vi "refmgr_register.vi"(8 "error in (no error)":errorcluster, 9 "ViName":string, 10 "VI Refnum":refnum<vi>, 11 "TagDB in":T1) -> (0 "error out":errorcluster, 2 "VI Refnum (dup)":refnum<vi>, 3 "TagDB out":T1)   [LabVIEW 2014, in "RefManager(dev).lvlib"]
uses:
  RefManager(dev).lvlib
  <userlib>/_NEVSTOP/TagDB/Core/tagDB_Def.ctl
  <userlib>/_NEVSTOP/TagDB/Core/TagDB.lvlib
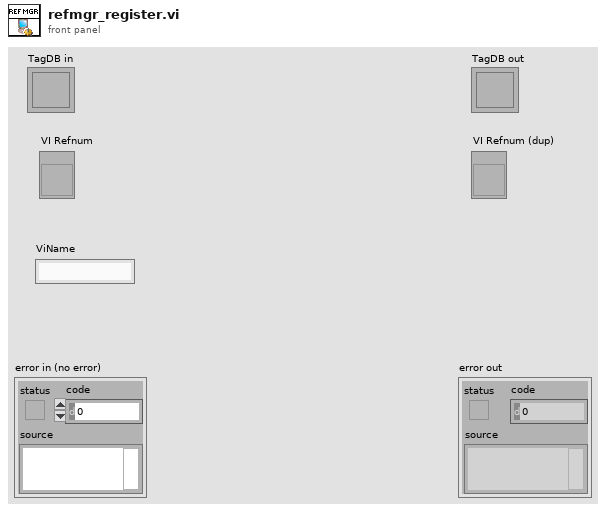
[diagram p1: front panel]
types:
  T1 = typedef "TagDB.lvlib/tagDB_Def.ctl" = refnum<k1>
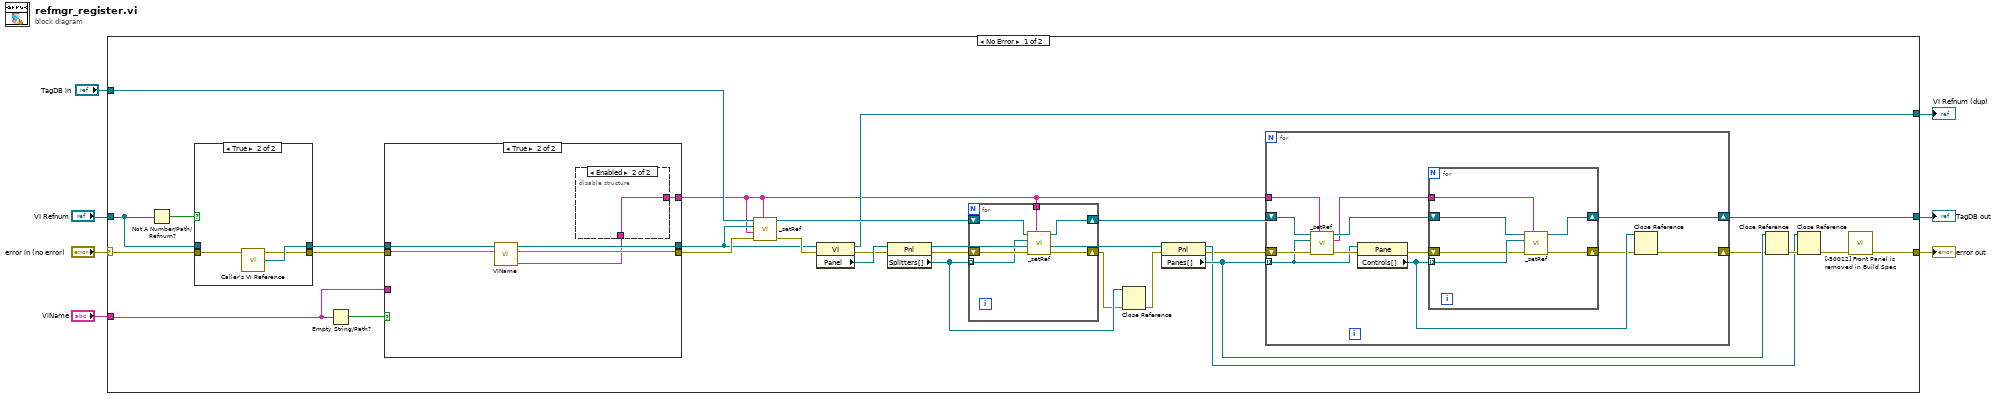
[diagram p0: block diagram]
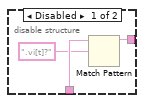
[diagram p3: hidden frame]
diagram:
  n1 = case shown="No Error" "error in (no error)" {
    selector: "error in (no error)" -> [w12 w82]
    tunnel: [w8 w82] -> w6
    tunnel: [w36 w81] -> w4
    tunnel: "TagDB in" -> [w16 w81]
    tunnel: "VI Refnum" -> [w33 w80]
    tunnel: "ViName" -> [w30 _]
    tunnel: [w14 w80] -> w1
    frame No Error {
      n2 = Not A Number/Path/Refnum?(number/path/refnum=w33) -> (NaN/Path/Refnum?=w13:bool)
      n3 = case shown="True" w13 {
        tunnel: w33 -> [w52 _]
        tunnel: [w52 w55] -> w32
        tunnel: w12 -> [w51 w53]
        tunnel: [w51 w54] -> w11
        frame False {
        }
        frame True {
          n4 = call "Caller's VI Reference.vi"("error in (no error)"=w53) -> ("error out"=w54:errorcluster, "Caller's VI Reference"=w55:refnum<vi>)  [unwired: 5 in]
        }
      }
      n5 = Empty String/Path?(string/path=w30) -> (empty?=w31:bool)
      n6 = case shown="True" w31 {
        tunnel: w32 -> [w39 w44]
        tunnel: [w39 w46] -> w17
        tunnel: w11 -> [w38 w43]
        tunnel: [w38 w42] -> w19
        tunnel: [w40 w45] -> w10
        tunnel: w30 -> [w40 _]
        frame False {
        }
        frame True {
          n7 = call "VIName.vi"("error in (no error)"=w43, "VI in"=w44) -> ("Name"=w41:string, "error out"=w42:errorcluster, "VI out"=w46:refnum<vi>)  [unwired: 7 in]
          n8 = disable-structure shown="Enabled" {
            disable-tunnel: w41 -> [w49 w50]
            disable-tunnel: [w48 w50] -> w45
            frame Disabled {
              n9 = Match Pattern(string=w49, regular expression=".vi[t]?") -> (before substring=w48:string)  [unwired: 1 in, 3 out]
            }
            frame Enabled {
            }
          }
        }
      }
      n10 = call "_setRef.vi"("parentURL"=w10, "error in (no error)"=w19, "Name"=w10, "Refnum"=w17, "TagDB in"=w16) -> ("error out"=w18:errorcluster, "TagDB out"=w15:T1)  [unwired: 4 in, 1 out]
      n11 = property class="VI"(reference=w17, error in=w18) -> (reference out=w14:refnum<vi>, error out=w26:errorcluster, "Panel"=w27:refnum<vi>)
      n12 = property class="Pnl"(reference=w27, error in=w26) -> (reference out=w25:refnum<vi>, error out=w23:errorcluster, "Splitters[]"=w22:refnum<vi>[])
      n13 = for {
        shift-right: [w59] -> w24
        shift-left: w15 -> [w60]
        tunnel: w22 -> [w57] mode=indexing
        shift-right: [w58] -> w21
        shift-left: w23 -> [w61]
        tunnel: w10 -> [w56]
        n14 = call "_setRef.vi"("parentURL"=w56, "error in (no error)"=w61, "Refnum"=w57, "TagDB in"=w60) -> ("error out"=w58:errorcluster, "TagDB out"=w59:T1)  [unwired: 5 in, 1 out]
      }
      n15 = Close Reference(reference=w22, error in (no error)=w21) -> (error out=w20:errorcluster)
      n16 = property class="Pnl"(reference=w25, error in=w20) -> (reference out=w29:refnum<vi>, error out=w28:errorcluster, "Panes[]"=w37:refnum<vi>[])
      n17 = for {
        tunnel: w37 -> [w64] mode=indexing
        shift-right: [w72] -> w36
        shift-left: w24 -> [w66]
        shift-right: [w69] -> w35
        shift-left: w28 -> [w68]
        tunnel: w10 -> [w63]
        n18 = call "_setRef.vi"("parentURL"=w63, "error in (no error)"=w68, "Refnum"=w64, "TagDB in"=w66) -> ("error out"=w67:errorcluster, "URL"=w62:string, "TagDB out"=w65:T1)  [unwired: 5 in]
        n19 = property class="Pane"(reference=w64, error in=w67) -> (error out=w71:errorcluster, "Controls[]"=w73:refnum<vi>[])  [unwired: 1 out]
        n20 = for {
          tunnel: w73 -> [w76] mode=indexing
          shift-right: [w78] -> w72
          shift-left: w65 -> [w79]
          shift-right: [w77] -> w70
          shift-left: w71 -> [w75]
          tunnel: w62 -> [w74]
          n21 = call "_setRef.vi"("parentURL"=w74, "error in (no error)"=w75, "Refnum"=w76, "TagDB in"=w79) -> ("error out"=w77:errorcluster, "TagDB out"=w78:T1)  [unwired: 5 in, 1 out]
        }
        n22 = Close Reference(reference=w73, error in (no error)=w70) -> (error out=w69:errorcluster)
      }
      n23 = Close Reference(reference=w37, error in (no error)=w35) -> (error out=w34:errorcluster)
      n24 = Close Reference(reference=w29, error in (no error)=w34) -> (error out=w9:errorcluster)
      n25 = call "[-50012] Front Panel is removed in Build Spec.vi"("error in (no error)"=w9) -> ("error out"=w8:errorcluster)  [unwired: 10 in]
    }
    frame Error {
    }
  }
  "error out" <- w6
  "TagDB out" <- w4
  "VI Refnum (dup)" <- w1
